vi "Visualize_exp.vi"(10 "ControlQueue":refnum<queue>, 11 "Message in":refnum<class "Message.lvclass">) -> ()   [LabVIEW 2018, in "Control-Client.lvclass"]
uses:
  Control-Client.lvclass
  Message/Message.lvclass
  controls/SliderSDII.ctl
  dependecies/ControlsVIs/Clusters-def/Standard Command.ctl
  dependecies/ControlsVIs/Clusters-def/Def_Vis_Addrow.ctl
  dependecies/ControlsVIs/Clusters-def/Def_Vis_Update.ctl
panel:
  out "wavelengths":dbl[](array[numeric])
  in  "times slider":T1={120.7741935483871, 734.8387096774194} scale=0.0..1.0 scale format="%#.1f"
  out "Spectra":cluster{"Y":dbl[], "Y":dbl[]}[](graph)
  in  "waves slider":T1={434.19354838709677, 734.8387096774194} scale=0.0..1.0 scale format="%#.1f"
  in  "LogY":bool
  out "Kinetics":cluster{"Y":dbl[], "Y":dbl[]}[](graph)
  out "Received command":string
  out "Exp data graph":dbl[][](graph)
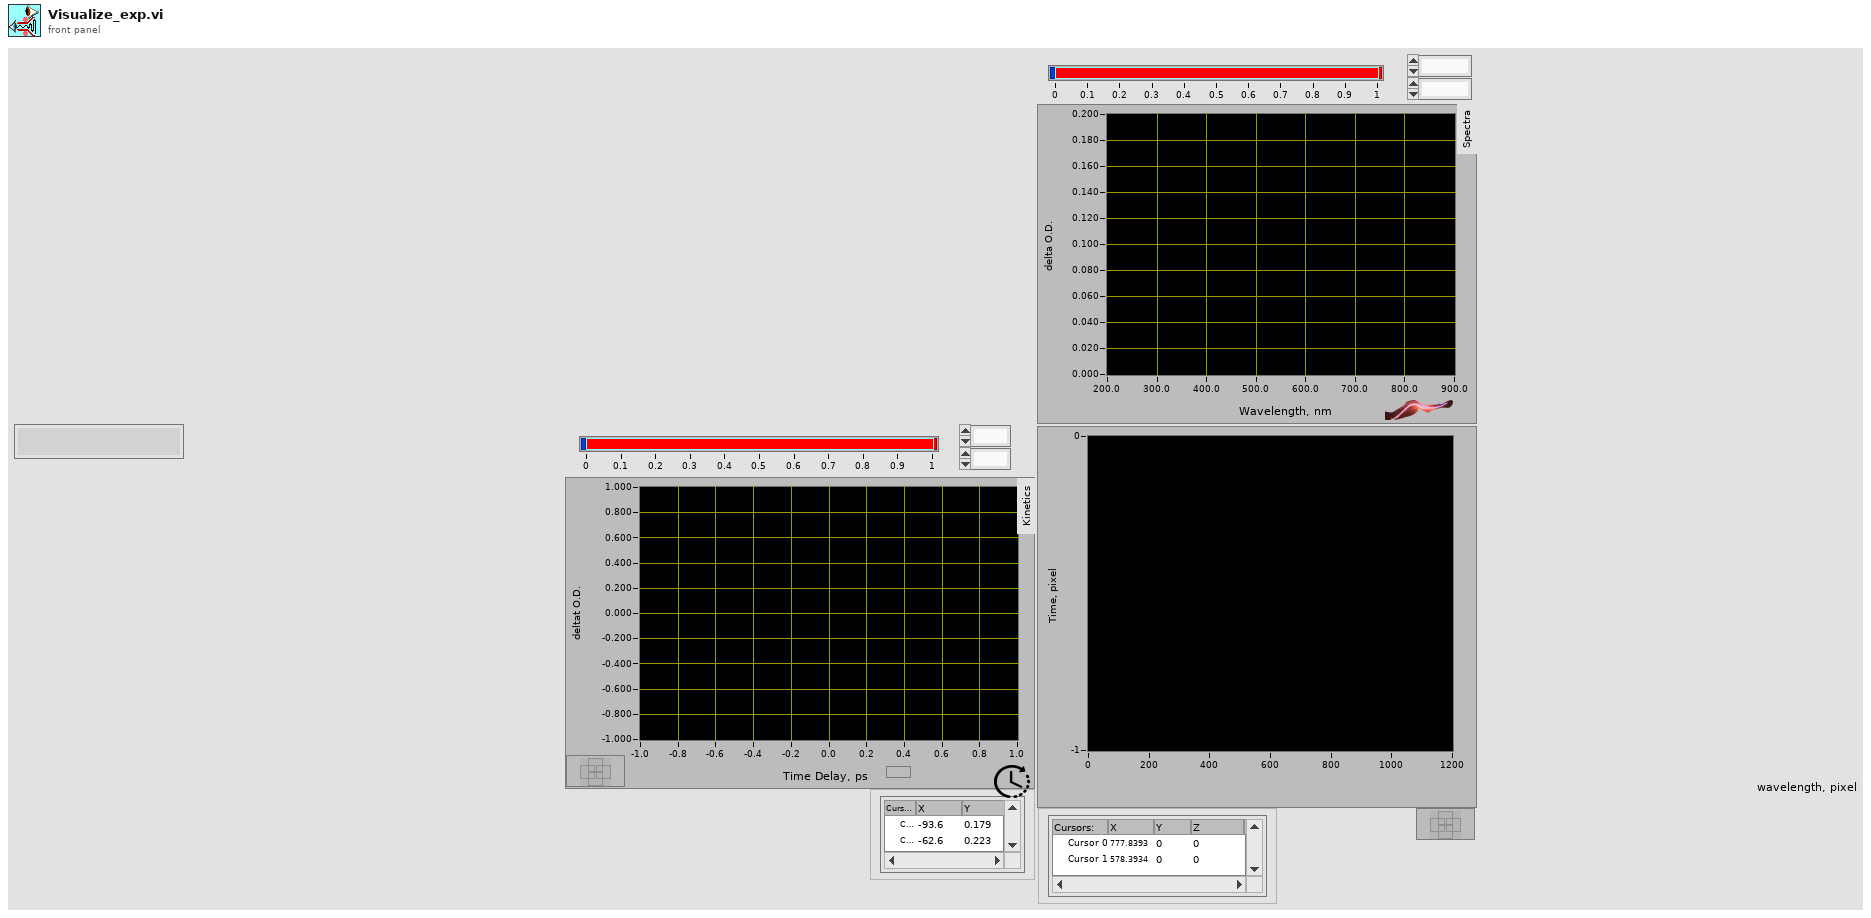
[diagram p1: front panel]
types:
  T1 = typedef "SliderSDII.ctl" = cluster{dbl, dbl}
  T2 = cluster{"times slider":refnum<vi>, "waves slider":refnum<vi>, "Kinetics":refnum<vi>, "Spectra":refnum<vi>, "Exp data graph":refnum<vi>}
  T3 = typedef "Standard Command.ctl" = cluster{"command":string, "data":variant}
  T4 = typedef "Control-Client.lvclass/Def_Vis_Addrow.ctl" = cluster{"row":sgl[], "timedelays":dbl[]}
  T5 = typedef "Control-Client.lvclass/Def_Vis_Update.ctl" = cluster{"Data":sgl[][], "timedelays":dbl[], "wavelength":dbl[]}
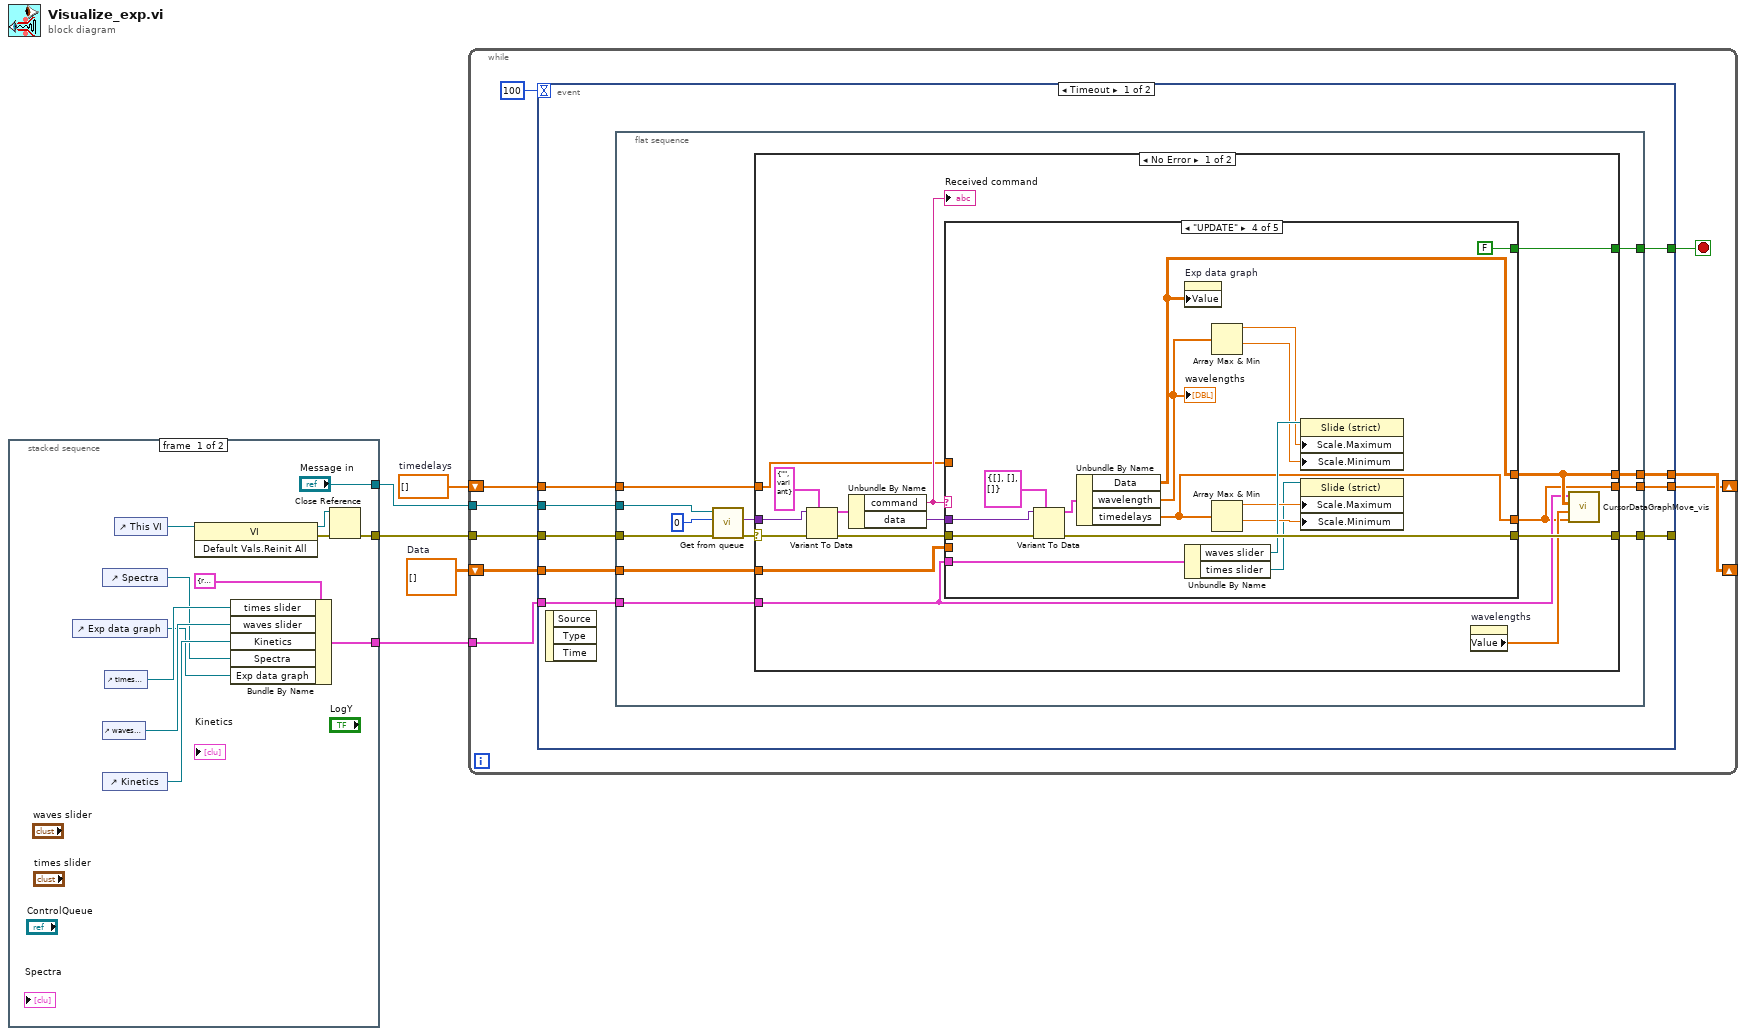
[diagram p0: block diagram]
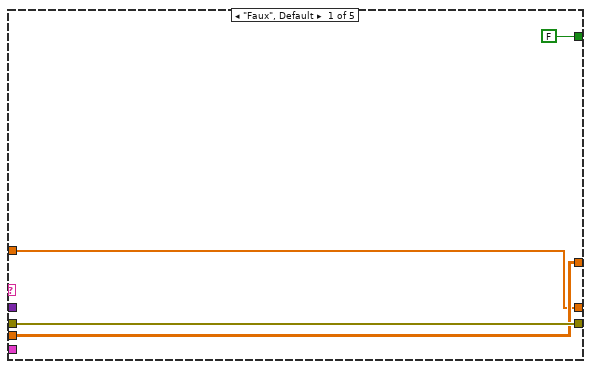
[diagram p3: hidden frame]
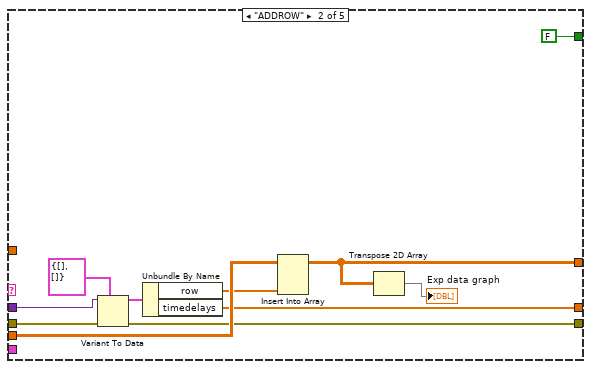
[diagram p4: hidden frame]
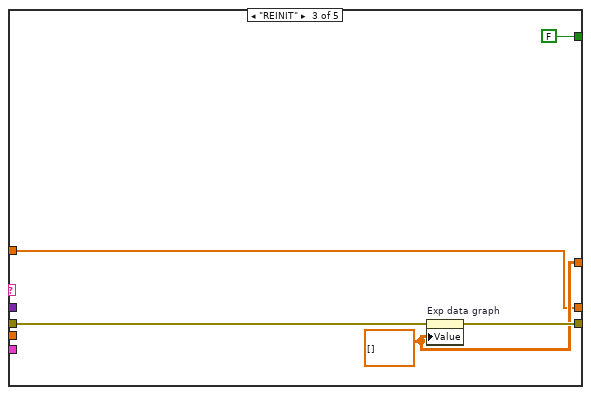
[diagram p5: hidden frame]
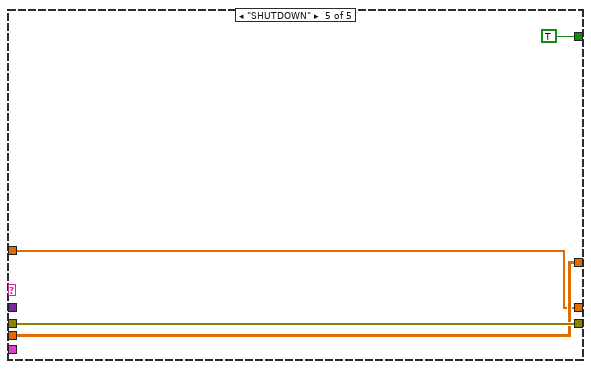
[diagram p6: hidden frame]
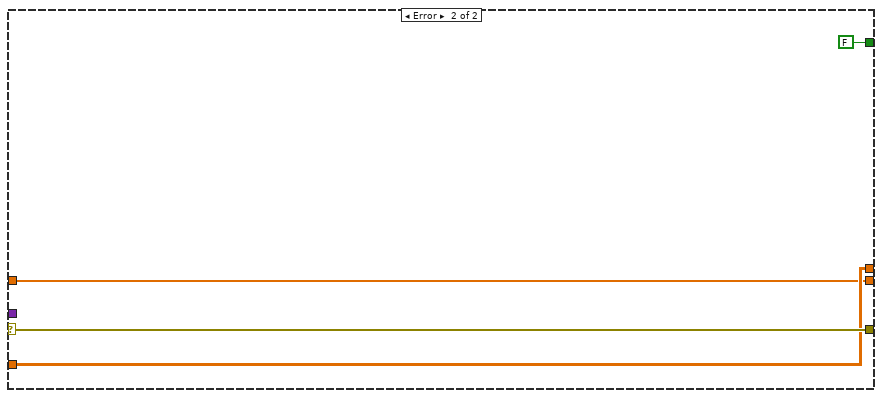
[diagram p7: hidden frame]
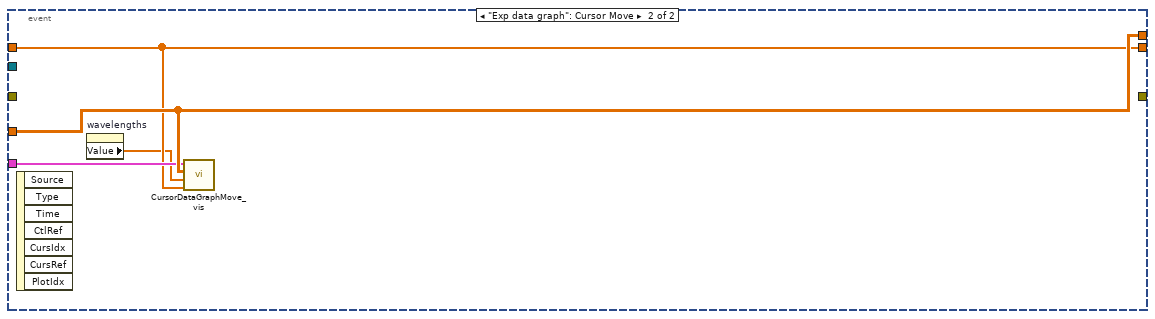
[diagram p8: hidden frame]
diagram:
  w1 = dbl[] []  # timedelays
  w3 = dbl[][] []  # Data
  n1 = stacked-sequence {
    tunnel: [w14 _] -> w5
    tunnel: ["Message in" _] -> w4
    tunnel: [w6 _] -> w2
    frame #0 {
      n2 = control-ref of="Exp data graph"() -> (w7:refnum<vi>)
      n3 = control-ref of="Spectra"() -> (w8:refnum<vi>)
      n4 = control-ref of="waves slider"() -> (w10:refnum<vi>)
      n5 = control-ref of="Kinetics"() -> (w9:refnum<vi>)
      n6 = control-ref of="times slider"() -> (w11:refnum<vi>)
      n7 = control-ref of="This VI"() -> (w15:refnum<vi>)
      n8 = invoke class="VI" method="Default Vals.Reinit All"(reference=w15) -> (reference out=w16:refnum<vi>, error out=w17:errorcluster)  [unwired: 2 in, 1 out]
      n9 = Bundle By Name(cluster=T2 {"times slider"=refnum, "waves slider"=refnum, "Kinetics"=refnum, "Spectra"=refnum, "Exp data graph"=refnum}, "times slider"=w11, "waves slider"=w10, "Kinetics"=w9, "Spectra"=w8, "Exp data graph"=w7) -> (w6:T2)
      n10 = Close Reference(reference=w16, error in (no error)=w17) -> (error out=w14:errorcluster)
    }
    frame #1 {
    }
  }
  n11 = while {
    tunnel: w5 -> [w24]
    tunnel: w4 -> [w23]
    shift-right: [w21] -> _
    shift-left: w3 -> [w22]
    tunnel: w2 -> [w20]
    shift-right: [w18] -> _
    shift-left: w1 -> [w19]
    stop <- w26 stop-if-true
    n12 = event shown="[0] Timeout" {
      selector: _ -> [_ _]
      dyn-events: _ -> [_ _]
      timeout: 100 -> [_ _]
      tunnel: [w34 _] -> _
      tunnel: [w35 _] -> w26
      tunnel: w24 -> [w33 _]
      tunnel: w23 -> [w32 _]
      tunnel: w22 -> [w31 w110]
      tunnel: [w30 w110] -> w21
      tunnel: w20 -> [w27 w109]
      tunnel: w19 -> [w29 w108]
      tunnel: [w28 w108] -> w18
      event Timeout {
        n13 = event-data() -> ()  [unwired: 1 in, 3 out]
        n14 = flat-sequence {
          tunnel: [w44] -> w35
          tunnel: [w43] -> w34
          tunnel: w33 -> [w41]
          tunnel: w32 -> [w42]
          tunnel: w31 -> [w40]
          tunnel: [w39] -> w30
          tunnel: w29 -> [w38]
          tunnel: [w37] -> w28
          tunnel: w27 -> [w36]
          frame #0 {
            n15 = call "Get from queue.vi"("error in (no error)"=w41, "timeout in ms (-1)"=0, "Message in"=w42) -> ("error out"=w45:errorcluster, "Data"=w46:variant)  [unwired: 5 in, 2 out]
            n16 = case shown="No Error" w45 {
              selector: w45 -> [w62 w105]
              tunnel: w46 -> [w57 _]
              tunnel: [w54 w105] -> w43
              tunnel: [w56 FALSE] -> w44
              tunnel: w40 -> [w53 w104]
              tunnel: [w51 w104] -> w39
              tunnel: w38 -> [w52 w103]
              tunnel: [w48 w103] -> w37
              tunnel: w36 -> [w50 _]
              frame No Error {
                n17 = Variant To Data(error in=w62, type=T3 {"command"="", "data"=variant} ("input cluster"), Variant=w57) -> (data=w60:T3, error out=w58:errorcluster)
                n18 = Unbundle By Name(w60) -> ("command"=w55:string, "data"=w59:variant)
                "Received command" <- w55
                n19 = case shown="\"UPDATE\"" w55 {
                  tunnel: [w66 w70 w81 w96 w101] -> w54
                  tunnel: [FALSE FALSE FALSE FALSE TRUE] -> w56
                  tunnel: w59 -> [_ w74 _ w98 _]
                  tunnel: w58 -> [w66 w76 w82 w97 w101]
                  tunnel: w53 -> [w64 w75 _ _ w100]
                  tunnel: [w64 w73 w79 w84 w100] -> w51
                  tunnel: w52 -> [w63 _ w78 _ w99]
                  tunnel: [w63 w67 w78 w83 w99] -> w48
                  tunnel: w50 -> [_ _ _ w92 _]
                  frame "Faux", Default {
                  }
                  frame "ADDROW" {
                    n20 = Variant To Data(error in=w76, type=T4 {"row"=[], "timedelays"=[]}, Variant=w74) -> (data=w69:T4, error out=w70:errorcluster)
                    n21 = Unbundle By Name(w69) -> ("row"=w68:sgl[], "timedelays"=w67:dbl[])
                    n22 = Insert Into Array(array=w75, new element=w68) -> (w73:dbl[][])  [unwired: 2 in]
                    n23 = Transpose 2D Array(2D array=w73) -> (transposed array=→"Exp data graph":dbl[][])
                  }
                  frame "REINIT" {
                    w79 = dbl[][] [] ("Exp data graph")
                    n24 = property on="Exp data graph" class="IntGraph (strict)"(error in=w82, "Value"=w79) -> (error out=w81:errorcluster)  [unwired: 1 in, 1 out]
                  }
                  frame "UPDATE" {
                    n25 = Variant To Data(error in=w97, type=T5 {"Data"=[], "timedelays"=[], "wavelength"=[]}, Variant=w98) -> (data=w93:T5, error out=w96:errorcluster)
                    n26 = Unbundle By Name(w93) -> ("Data"=w84:sgl[][], "wavelength"=w90:dbl[], "timedelays"=w83:dbl[])
                    "wavelengths" <- w90
                    n27 = property on="Exp data graph" class="IntGraph (strict)"("Value"=w84) -> ()  [unwired: 2 in, 2 out]
                    n28 = Unbundle By Name(w92) -> ("waves slider"=w91:refnum<vi>, "times slider"=w85:refnum<vi>)
                    n29 = Array Max & Min(array=w90) -> (max value=w89:dbl, min value=w88:dbl)  [unwired: 2 out]
                    n30 = Array Max & Min(array=w83) -> (max value=w87:dbl, min value=w86:dbl)  [unwired: 2 out]
                    n31 = property class="Slide (strict)"(reference=w91, "Scale.Maximum"=w89, "Scale.Minimum"=w88) -> ()  [unwired: 1 in, 2 out]
                    n32 = property class="Slide (strict)"(reference=w85, "Scale.Maximum"=w87, "Scale.Minimum"=w86) -> ()  [unwired: 1 in, 2 out]
                  }
                  frame "SHUTDOWN" {
                  }
                }
                n33 = property on="wavelengths" class="Arr (strict)"() -> ("Value"=w49:dbl[])  [unwired: 2 in, 2 out]
                n34 = call "CursorDataGraphMove_vis.vi"("timedelays"=w48, "wavelengths"=w49, "Data"=w51, "References"=w50) -> ()  [unwired: 4 in]
              }
              frame Error {
              }
            }
          }
        }
      }
      event "Exp data graph": Cursor Move {
        n35 = event-data() -> ()  [unwired: 1 in, 7 out]
        n36 = property on="wavelengths" class="Arr (strict)"() -> ("Value"=w107:dbl[])  [unwired: 2 in, 2 out]
        n37 = call "CursorDataGraphMove_vis.vi"("timedelays"=w108, "wavelengths"=w107, "Data"=w110, "References"=w109) -> ()  [unwired: 4 in]
      }
    }
  }
